vi "Tray_TrayDataToUI.vi"(0 "TrayInRefIn":refnum<vi>, 5 "Tray":bool[][](array[boolean]), 7 "TrayType":T1, 9 "TraySize":cluster{"y":u32, "x":u32}={"y"=16, "x"=6}, 11 "error in":errorcluster) -> (15 "error out":errorcluster)   [LabVIEW 2014]
uses:
  Tray_TrayName.ctl
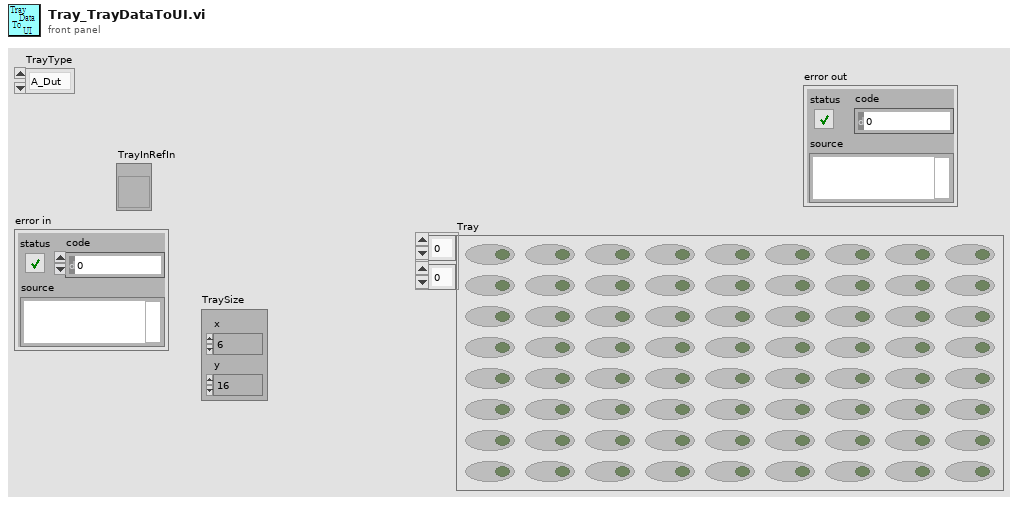
[diagram p1: front panel]
types:
  T1 = typedef "Tray_TrayName.ctl" = enum16{"A_Dut", "B_Pass", "C_NGL", "D_NGR"}
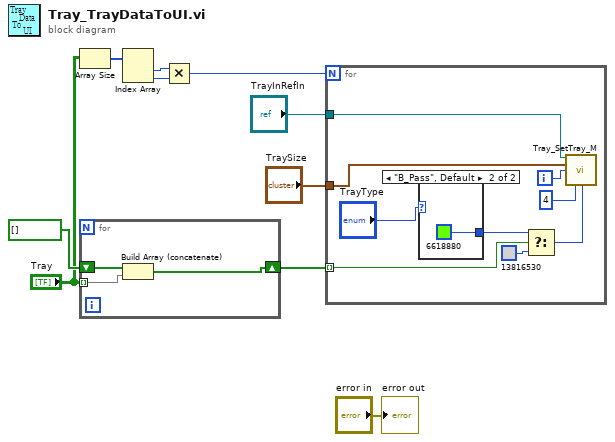
[diagram p0: block diagram]
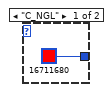
[diagram p2: hidden frame]
diagram:
  n1 = Array Size(array="Tray") -> (size(s)=w4:i32[])
  n2 = for {
    tunnel: "Tray" -> [w12] mode=indexing
    shift-right: [w11] -> w10
    shift-left: bool[] [] ("DutTray") -> [w13]
    n3 = Build Array (concatenate)(w13, w12) -> (w11:bool[])
  }
  n4 = Index Array(array=w4) -> (element #1=w5:i32, element #2=w6:i32)  [unwired: 2 in]
  n5 = Multiply(x=w5, y=w6) -> (x*y=w7:i32)
  n6 = for {
    N: w7 -> [_]
    tunnel: w10 -> [w21] mode=indexing
    tunnel: "TrayInRefIn" -> [w16]
    tunnel: "TraySize" -> [w15]
    i -> [w20]
    n7 = case shown="\"B_Pass\", Default" "TrayType" {
      tunnel: [u32 16711680 ("Initial color") u32 6618880 ("Initial color")] -> w18
      frame "C_NGL" {
      }
      frame "B_Pass", Default {
      }
    }
    n8 = Select(t=w18, s=w21, f=u32 13816530 ("Initial color")) -> (s? t:f=w17:u32)
    n9 = call "Tray_SetTray_M.vi"("TrayIn"=w16, "GridSize"=w15, "Index Number"=w20, "Direction"=u16 4, "Color Box"=w17) -> ()  [unwired: 10 in, 1 out]
  }
  "error out" <- "error in"
